vi "2_3_Procesos.vi"() -> ()   [LabVIEW 2020]
panel:
  out "x = y? 2":bool
  in  "y 2":i32
  in  "y":i32
  out "x = y?":bool
  out "TANQUE":dbl(slide) scale=0.0..10.0
  out "TERMOMETRO":dbl(slide) scale=25.0..90.0
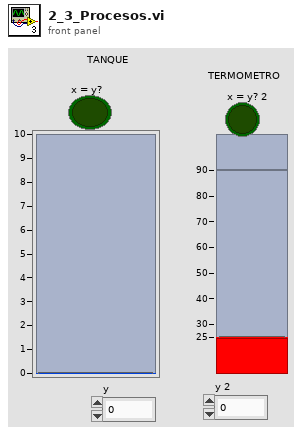
[diagram p1: front panel]
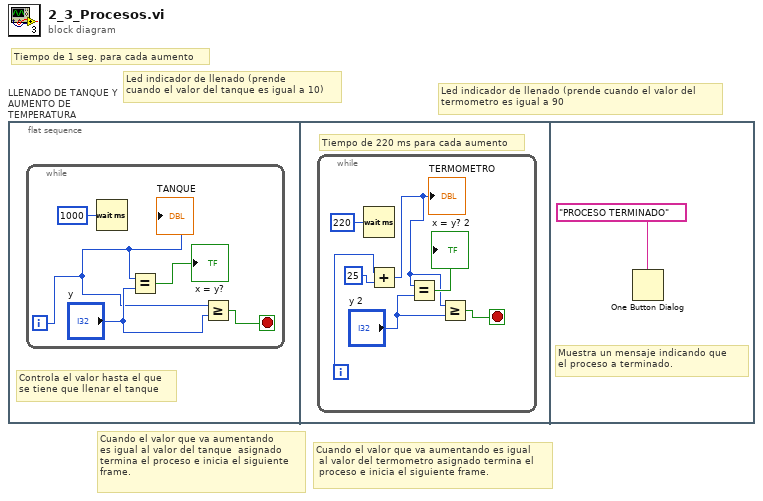
[diagram p0: block diagram]
diagram:
  # "Cuando el valor que va aumentando es igual\n al valor del termometro asignado termina el\n proceso e inicia el siguiente frame."
  # "Led indicador de llenado (prende cuando el valor del \ntermometro es igual a 90"
  # "Cuando el valor que va aumentando \nes igual al valor del tanque  asignado \ntermina el proceso e inicia el siguiente \nframe."
  # "Led indicador de llenado (prende \ncuando el valor del tanque es igual a 10)"
  # "Tiempo de 1 seg. para cada aumento"
  n1 = flat-sequence "LLENADO DE TANQUE Y AUMENTO DE TEMPERATURA" {
    frame #0 {
      # "Controla el valor hasta el que \nse tiene que llenar el tanque"
      n2 = while {
        i -> [w1]
        stop <- w3 stop-if-true
        n3 = Wait (ms)(milliseconds to wait=u32 1000) -> ()  [unwired: 1 out]
        n4 = Equal?(x=w1, y="y") -> (x = y?=→"x = y?":bool)
        n5 = Greater Or Equal?(x=w1, y="y") -> (x >= y?=w3:bool)
        "TANQUE" <- w1
      }
    }
    frame #1 {
      # "Tiempo de 220 ms para cada aumento"
      n6 = while {
        i -> [w7]
        stop <- w10 stop-if-true
        n7 = Wait (ms)(milliseconds to wait=u32 220) -> ()  [unwired: 1 out]
        n8 = Add(x=w7, y=25) -> (x+y=w6:i32)
        "TERMOMETRO" <- w6
        n9 = Equal?(x=w6, y="y 2") -> (x = y?=→"x = y? 2":bool)
        n10 = Greater Or Equal?(x=w6, y="y 2") -> (x >= y?=w10:bool)
      }
    }
    frame #2 {
      # "Muestra un mensaje indicando que \nel proceso a terminado."
      n11 = One Button Dialog(message="PROCESO TERMINADO") -> ()  [unwired: 1 in, 1 out]
    }
  }
